vi "Get Server Stop UE.vi"(11 "OOP Server in":refnum<class "TestDataMarshal.lvclass">) -> (2 "Server Stop":refnum<user-event>, 3 "OOP Server out":refnum<class "TestDataMarshal.lvclass">)   [LabVIEW 2019, in "TestDataMarshal.lvlib" / "TestDataMarshal.lvclass"]
uses:
  TestDataMarshal.lvclass
  TestDataMarshal.lvclass/TestDataMarshal.ctl
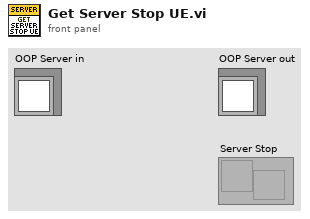
[diagram p1: front panel]
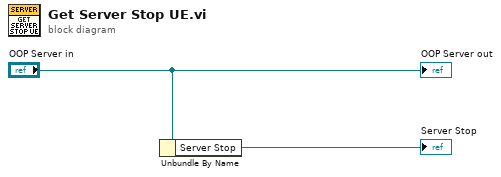
[diagram p0: block diagram]
diagram:
  n1 = Unbundle By Name("OOP Server in") -> ("Server Stop"=→"Server Stop":refnum<user-event>)
  "OOP Server out" <- "OOP Server in"
